vi "ADIS16448 Config Cal Time.vi"(8 "error in (no error)":errorcluster, 9 "Data":u32, 10 "timeout in ms (-1)":i32, 11 "ADIS16448DevRef in":T1={"DevStatus"={"status"=FALSE, "code"=0, "source"=""}, "Hardware Config"={"SPI Clock Rate (Hz)"=0.0, "IMU SPI Mode (3)"=enum."Mode 0 (Clk Idle Low,Sample on Leading)", "IMU Reset Pin"=enum."DIO 0", "IMU SPI Bus"=enum."SPI On-Board, CS0", "IMU Data Ready Pin"=enum."DIO 0", "Stall Config"={"Pow2BytesPerRead"=255, "StallTicks"=640, "CsToSclkTicks"=5}, "IMU Status LED Pin"=enum."DIO MXP 9"}, "Calibration Complete"=refnum, "Status FIFO"=refnum, "Last Value Reference"=refnum, "Sychronous Process VI"=refnum, "Cmd FIFO"=refnum, "Source"={"DevStatus"={"status"=FALSE, "code"=0, "source"=""}, "AnalogTriggerMode?"=FALSE, "DigitalMode"={"DIO Channel"=enum."Disabled"}, "AnalogTriggerMode"={"AnalogTriggerIndex"=enum."Trig 0", "OutputType"=enum."InWindow"}}, "Data FIFO"=refnum, "IMU Status LED Pin"=enum."DIO MXP 9", "Calibration Time"=5}) -> (0 "error out":errorcluster, 3 "ADIS16448DevRef out":T1={"DevStatus"={"status"=FALSE, "code"=0, "source"=""}, "Hardware Config"={"SPI Clock Rate (Hz)"=0.0, "IMU SPI Mode (3)"=enum."Mode 0 (Clk Idle Low,Sample on Leading)", "IMU Reset Pin"=enum."DIO 0", "IMU SPI Bus"=enum."SPI On-Board, CS0", "IMU Data Ready Pin"=enum."DIO 0", "Stall Config"={"Pow2BytesPerRead"=255, "StallTicks"=640, "CsToSclkTicks"=5}, "IMU Status LED Pin"=enum."DIO MXP 9"}, "Calibration Complete"=refnum, "Status FIFO"=refnum, "Last Value Reference"=refnum, "Sychronous Process VI"=refnum, "Cmd FIFO"=refnum, "Source"={"DevStatus"={"status"=FALSE, "code"=0, "source"=""}, "AnalogTriggerMode?"=FALSE, "DigitalMode"={"DIO Channel"=enum."Disabled"}, "AnalogTriggerMode"={"AnalogTriggerIndex"=enum."Trig 0", "OutputType"=enum."InWindow"}}, "Data FIFO"=refnum, "IMU Status LED Pin"=enum."DIO MXP 9", "Calibration Time"=5})   [LabVIEW 2019]
doc: "This VI triggers a re-calibration routine on the ADIS16470. This call will take approx. 100ms to run. The sensor <b><u>MUST</b></u> be completely still before calling this method. To set the amount of time before this call to calibrate call <b>ADIS16470 Set Re-calibration Time</b>. The default is ~1s.\n\nA good use for this is to set the calibration time so a reasonable amount of time that the robot may be still (for example, while the robot is on the field before Autonomous). Then call this routine at the start of autonomous to set good calibration. The sensor uses the samples before this method is called in its calibration. The longer the time the better the result, though the improvement is lower after 8s-16s."
uses:
  Typedef/ADIS16448 Device Reference.ctl
  Typedef/ADIS16448 Hardware Configuration.ctl
  <vilib>/Rock Robotics/WPI/SPI/WPI_SPIMode.ctl
  <vilib>/Rock Robotics/SystemInterfaces/DIO/FPGA_DIOChannel.ctl
  <vilib>/Rock Robotics/SystemInterfaces/spilib/spi_bus.ctl
  Typedef/ADIS16448 Status.ctl
  Typedef/ADIS16448 Data.ctl
  Typedef/ADIS16448 Process.ctl
  Typedef/ADIS16448 Command Type.ctl
  <vilib>/Rock Robotics/SystemInterfaces/CounterEncoderSourceConvertion/FPGA_CounterEncoderSourceConvertionLVSourceType.ctl
  <vilib>/Rock Robotics/SystemInterfaces/DIO/FPGA_DIODigitalSourceChannel.ctl
  <vilib>/Rock Robotics/SystemInterfaces/AnalogTrigger/FPGA_AnalogTriggerIndex.ctl
  <vilib>/Rock Robotics/SystemInterfaces/AnalogTrigger/FPGA_AnalogTriggerOutType.ctl
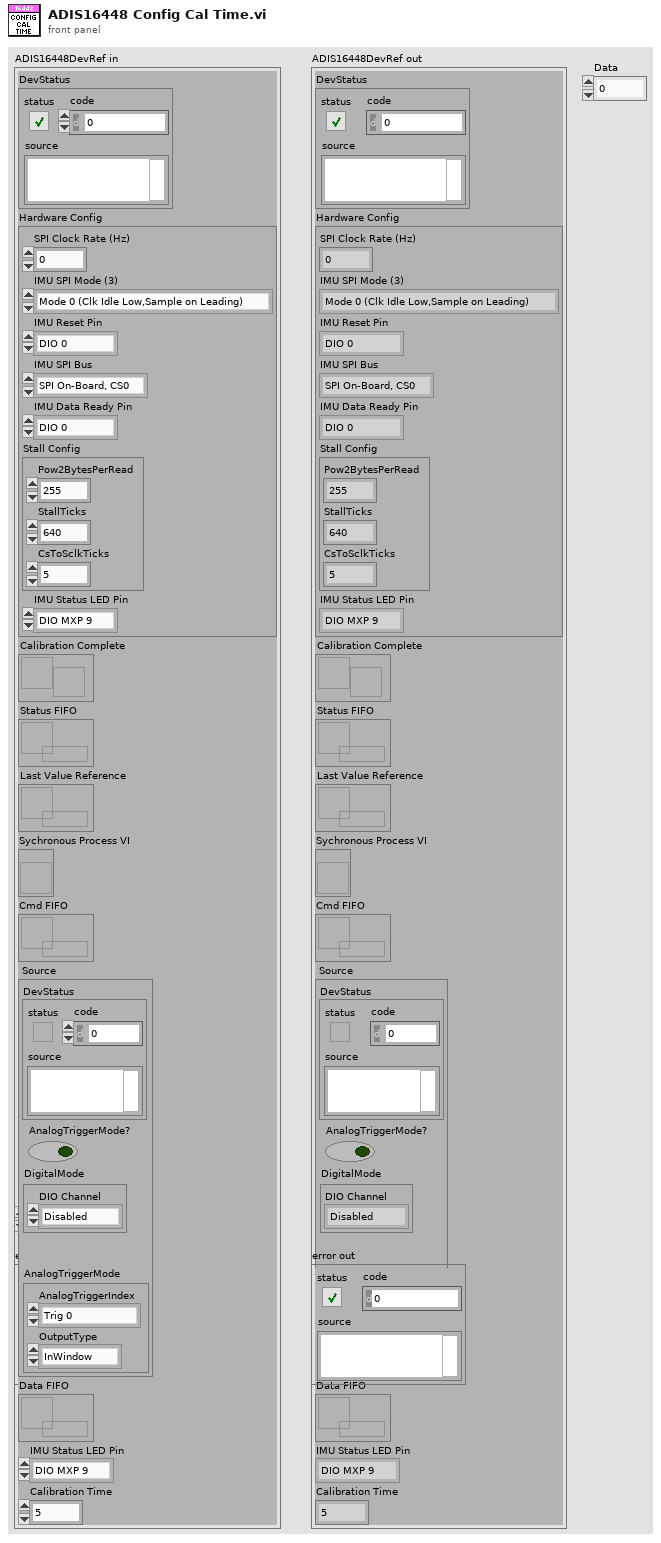
[diagram p1: front panel]
types:
  T1 = typedef "ADIS16448 Device Reference.ctl" = cluster{"DevStatus":errorcluster, "Hardware Config":T2, "Calibration Complete":refnum<notifier>, "Status FIFO":refnum<k33>, "Last Value Reference":refnum<data-value>, "Sychronous Process VI":T6, "Cmd FIFO":refnum<k33>, "Source":T7, "Data FIFO":refnum<k33>, "IMU Status LED Pin":T4, "Calibration Time":u32}
  T2 = typedef "ADIS16448 Hardware Configuration.ctl" = cluster{"SPI Clock Rate (Hz)":dbl, "IMU SPI Mode (3)":T3, "IMU Reset Pin":T4, "IMU SPI Bus":T5, "IMU Data Ready Pin":T4, "Stall Config":cluster{"Pow2BytesPerRead":u8, "StallTicks":u16, "CsToSclkTicks":u8}, "IMU Status LED Pin":T4}
  T3 = typedef "WPI_SPIMode.ctl" = enum16{"Mode 0 (Clk Idle Low,Sample on Leading)", "Mode 1 (Clk Idle Low,Sample on Trailing)", "Mode 2 (Clk Idle High,Sample on Leading)", "Mode 3 (Clk Idle High,Sample on Trailing)"}
  T4 = typedef "FPGA_DIOChannel.ctl" = enum8{"DIO 0", "DIO 1", "DIO 2", "DIO 3", "DIO 4", "DIO 5", "DIO 6", "DIO 7", "DIO 8", "DIO 9", "DIO MXP 0", "DIO MXP 1", "DIO MXP 2", "DIO MXP 3", "DIO MXP 4", "DIO MXP 5", "DIO MXP 6", "DIO MXP 7", "DIO MXP 8", "DIO MXP 9", "DIO MXP 10", "DIO MXP 11", "DIO MXP 12", "DIO MXP 13", "DIO MXP 14", "DIO MXP 15", "SPI Port CS1", "SPI Port CS2", "SPI Port CS3", "SPI Port MISO", "SPI Port MOSI", "Invalid"}
  T5 = typedef "spi_bus.ctl" = enum16{"SPI On-Board, CS0", "SPI On-Board, CS1", "SPI On-Board, CS2", "SPI On-Board, CS3", "SPI MXP", "Invalid"}
  T6 = typedef "ADIS16448 Process.ctl" = refnum<vi>
  T7 = typedef "FPGA_CounterEncoderSourceConvertionLVSourceType.ctl" = cluster{"DevStatus":errorcluster, "AnalogTriggerMode?":bool, "DigitalMode":cluster{"DIO Channel":T8}, "AnalogTriggerMode":cluster{"AnalogTriggerIndex":T9, "OutputType":T10}}
  T8 = typedef "FPGA_DIODigitalSourceChannel.ctl" = enum8{"DIO 0", "DIO 1", "DIO 2", "DIO 3", "DIO 4", "DIO 5", "DIO 6", "DIO 7", "DIO 8", "DIO 9", "DIO MXP 0", "DIO MXP 1", "DIO MXP 2", "DIO MXP 3", "DIO MXP 4", "DIO MXP 5", "DIO MXP 6", "DIO MXP 7", "DIO MXP 8", "DIO MXP 9", "DIO MXP 10", "DIO MXP 11", "DIO MXP 12", "DIO MXP 13", "DIO MXP 14", "DIO MXP 15", "SPI Port CS1", "SPI Port CS2", "SPI Port CS3", "SPI Port MISO", "SPI Port MOSI", "Disabled"}
  T9 = typedef "FPGA_AnalogTriggerIndex.ctl" = enum8{"Trig 0", "Trig 1", "Trig 2", "Trig 3", "Trig 4", "Trig 5", "Trig 6", "Trig 7", "Invalid"}
  T10 = typedef "FPGA_AnalogTriggerOutType.ctl" = enum16{"InWindow", "TriggerState", "Rising", "Falling"}
  T11 = enum16{"None", "Reset", "Rewrite Config", "Start Recal", "Recalibrate", "Recal Complete", "Exit Auto SPI", "Start Auto SPI", "Configure Cal"}
  T12 = typedef "ADIS16448 Command Type.ctl" = cluster{"Command":enum16{"None", "Reset", "Rewrite Config", "Start Recal", "Recalibrate", "Recal Complete", "Exit Auto SPI", "Start Auto SPI", "Configure Cal"}, "Data":u32}
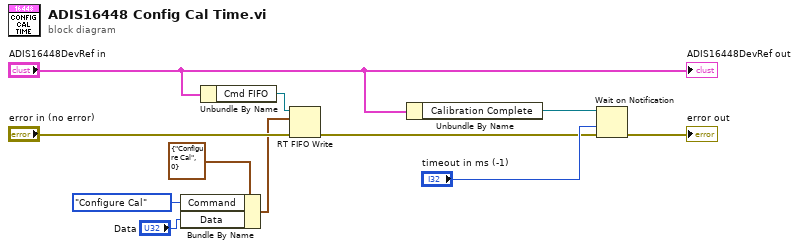
[diagram p0: block diagram]
diagram:
  n1 = Bundle By Name(cluster=T12 {"Command"=enum."Configure Cal", "Data"=0} ("Input"), "Command"=T11."Configure Cal", "Data"="Data") -> (w3:T12)
  n2 = Unbundle By Name("ADIS16448DevRef in") -> ("Cmd FIFO"=w8:refnum<k33>)
  n3 = RT FIFO Write(0:w8, 1:w3, 3:"error in (no error)") -> (11:w5:errorcluster)  [unwired: 2 in, 3 out]
  n4 = Unbundle By Name("ADIS16448DevRef in") -> ("Calibration Complete"=w10:refnum<notifier>)
  n5 = Wait on Notification(notifier=w10, timeout in ms (-1)="timeout in ms (-1)", error in (no error)=w5) -> (error out=→"error out":errorcluster)  [unwired: 1 in, 3 out]
  "ADIS16448DevRef out" <- "ADIS16448DevRef in"
